vi "WebServiceImporter Reference.vi"(8 "error in (no error)":errorcluster, 9 "Operation":enum16{"Get", "Set"}(ring), 11 "Web Service Importer":refnum<k24>) -> (0 "error out":errorcluster, 3 "Web Service Importer out":refnum<k24>)   [LabVIEW 2017, in "WebServiceImporter.lvlib" / "ProxyDll Generator.lvlib"]
uses:
  <vilib>/Platform/WebService/ProxyDll Generator/ProxyDll Generator.lvlib
  e:/builds/penguin/labview/branches/2017/dev/dist/resource/WebServiceUtils.dll
  resource/WebServiceUtils.dll
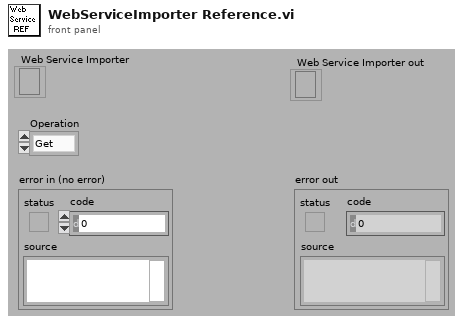
[diagram p1: front panel]
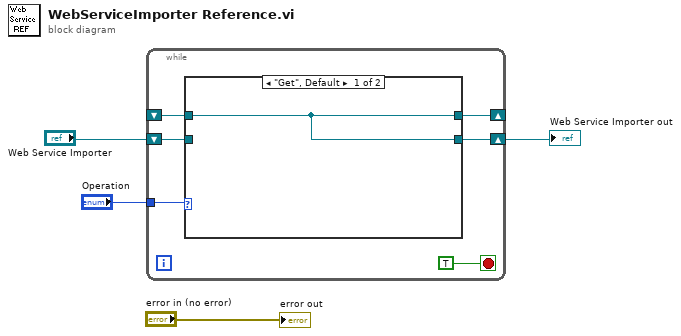
[diagram p0: block diagram]
diagram:
  n1 = while {
    tunnel: "Operation" -> [w10]
    shift-right: [w8] -> w3
    shift-left: "Web Service Importer" -> [w9]
    shift-right: [w7] -> _
    shift-left: _ -> [w6]
    stop <- TRUE stop-if-true
    n2 = case shown="\"Get\", Default" w10 {
      tunnel: w9 -> [_ w12]
      tunnel: [w11 w12] -> w8
      tunnel: [w11 w12] -> w7
      tunnel: w6 -> [w11 _]
      frame "Get", Default {
      }
      frame "Set" {
      }
    }
  }
  "Web Service Importer out" <- w3
  "error out" <- "error in (no error)"
